vi "get_number_neighbours.vi"(8 "index2":dbl, 9 "index1":dbl, 11 "Array":dbl[][](array[numeric])) -> (1 "Numeric":i32)   [LabVIEW 2016]
panel:
  out "Array 3":dbl[](array[numeric])
  out "Array 2":cluster{"outdex1":dbl, "outdex2":dbl}[](array[cluster])
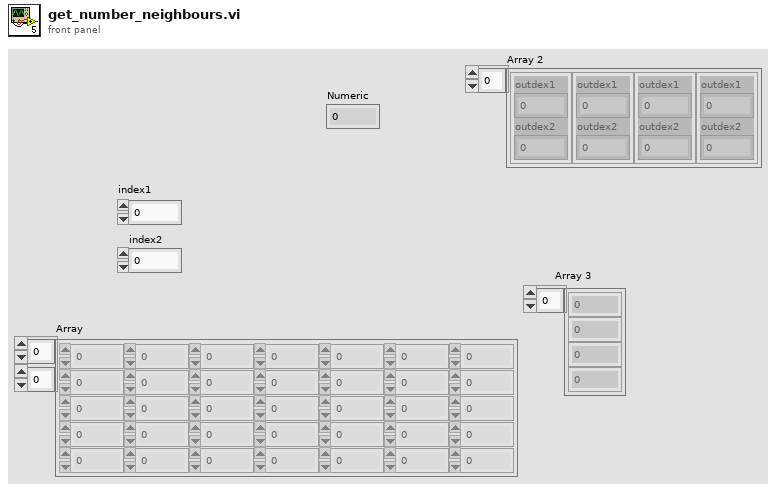
[diagram p1: front panel]
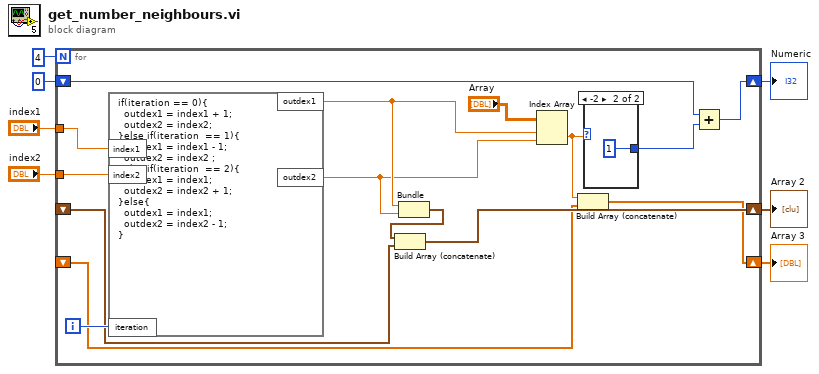
[diagram p0: block diagram]
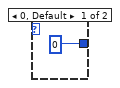
[diagram p2: hidden frame]
diagram:
  n1 = for {
    N: 4 -> [_]
    shift-right: [w16] -> w3
    shift-left: 0 -> [w17]
    tunnel: "index1" -> [w22]
    tunnel: "index2" -> [w21]
    shift-right: [w11] -> w2
    shift-left: _ -> [w13]
    shift-right: [w9] -> w1
    shift-left: _ -> [w8]
    i -> [w20]
    n2 = formula code="if(iteration == 0){\n  outdex1 = index1 + 1;\n  outdex2 = index2;\n}else if(iteration  == 1){\n  outdex1 = index1 - 1;\n  outdex2 = index2 ;\n}else if(iteration  == 2){\n  outdex1 = index1;\n  outdex2 = index2 + 1;\n}else{\n  outdex1 = index1;\n  outdex2 = index2 - 1;\n}"("index1"=w22, "index2"=w21, "iteration"=w20) -> ("outdex1"=w15:dbl, "outdex2"=w14:dbl)
    n3 = Bundle("outdex1"=w15, "outdex2"=w14) -> (w12:cluster{"outdex1":dbl, "outdex2":dbl})  [unwired: 1 in]
    n4 = Build Array (concatenate)(w12, w13) -> (w11:cluster{"outdex1":dbl, "outdex2":dbl}[])
    n5 = Index Array(array="Array", index (row)=w15, index (col)=w14) -> (element=w10:dbl)
    n6 = Build Array (concatenate)(w10, w8) -> (w9:dbl[])
    n7 = case shown="-2" w10 {
      tunnel: [0 1] -> w18
      frame 0, Default {
      }
      frame -2 {
      }
    }
    n8 = Add(x=w17, y=w18) -> (x+y=w16:i32)
  }
  "Numeric" <- w3
  "Array 2" <- w2
  "Array 3" <- w1
